vi "DAQGlobal.vi"() -> ()   [LabVIEW 2009]
panel:
  in  "Saving?":bool
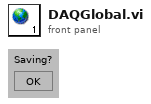
[diagram p1: front panel]
diagram:
